vi "Test Matrix Mult.vi"() -> ()   [LabVIEW 2014, in "Arduino MatrixMath.lvlib"]
uses:
  <vilib>/Aledyne-TSXperts/Arduino Compatible Compiler for LabVIEW/addons/Arduino MatrixMath/Arduino MatrixMath.lvlib
panel:
  in  "B":sgl[](array[numeric])
  in  "A":sgl[](array[numeric])
  out "A*B":sgl[](array[numeric])
  out "Error Out":errorcluster
  in  "Error In":errorcluster
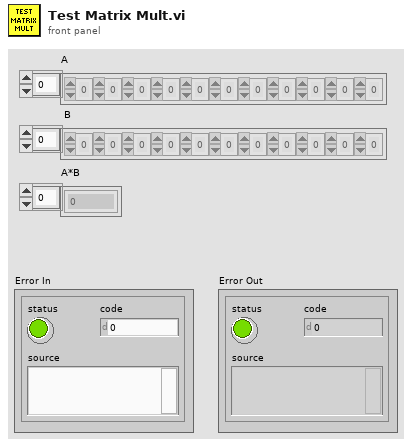
[diagram p1: front panel]
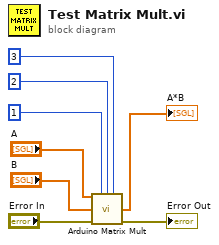
[diagram p0: block diagram]
diagram:
  n1 = call <vilib>:"Arduino Matrix Mult.vi"("A"="A", "A rows"=u8 1, "A cols = B rows"=u8 2, "B cols"=u8 3, "B"="B", "Error In"="Error In") -> ("A*B"=→"A*B":sgl[], "Error Out"=→"Error Out":errorcluster)  [unwired: 8 in]
